vi "wifi-sub.vi"(0 "IP address":refnum<visa-resource-name>="COM13", 1 "send data":string, 5 "error in (no error)":errorcluster, 6 "port":i32, 7 "timeout (10sec)":u32=10000, 9 "data存盘":bool=TRUE, 10 "mode":T1(ring), 11 "Receive bytes one time":i32=1452) -> (15 "timeout?":bool=TRUE, 19 "error IO":errorcluster)   [LabVIEW 2023, in "wifi-interface.lvlib"]
uses:
  wifi-interface.lvlib
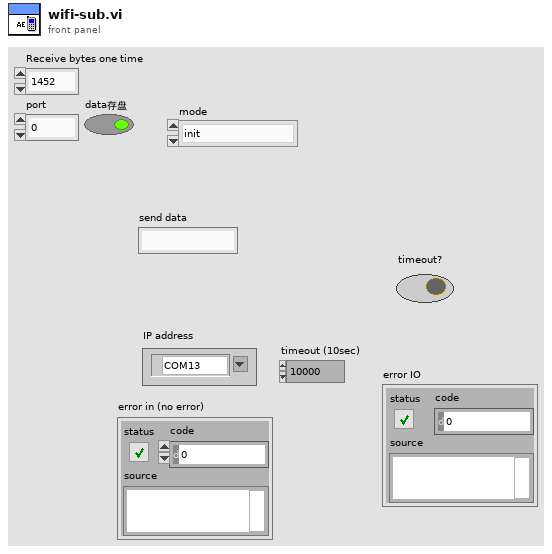
[diagram p1: front panel]
types:
  T1 = enum16{"init", "broadcast_data", "receive_data", "close", "clear_visa"}
  T2 = enum16{"Standard", "Buffered", "CRLF", "Immediate"}
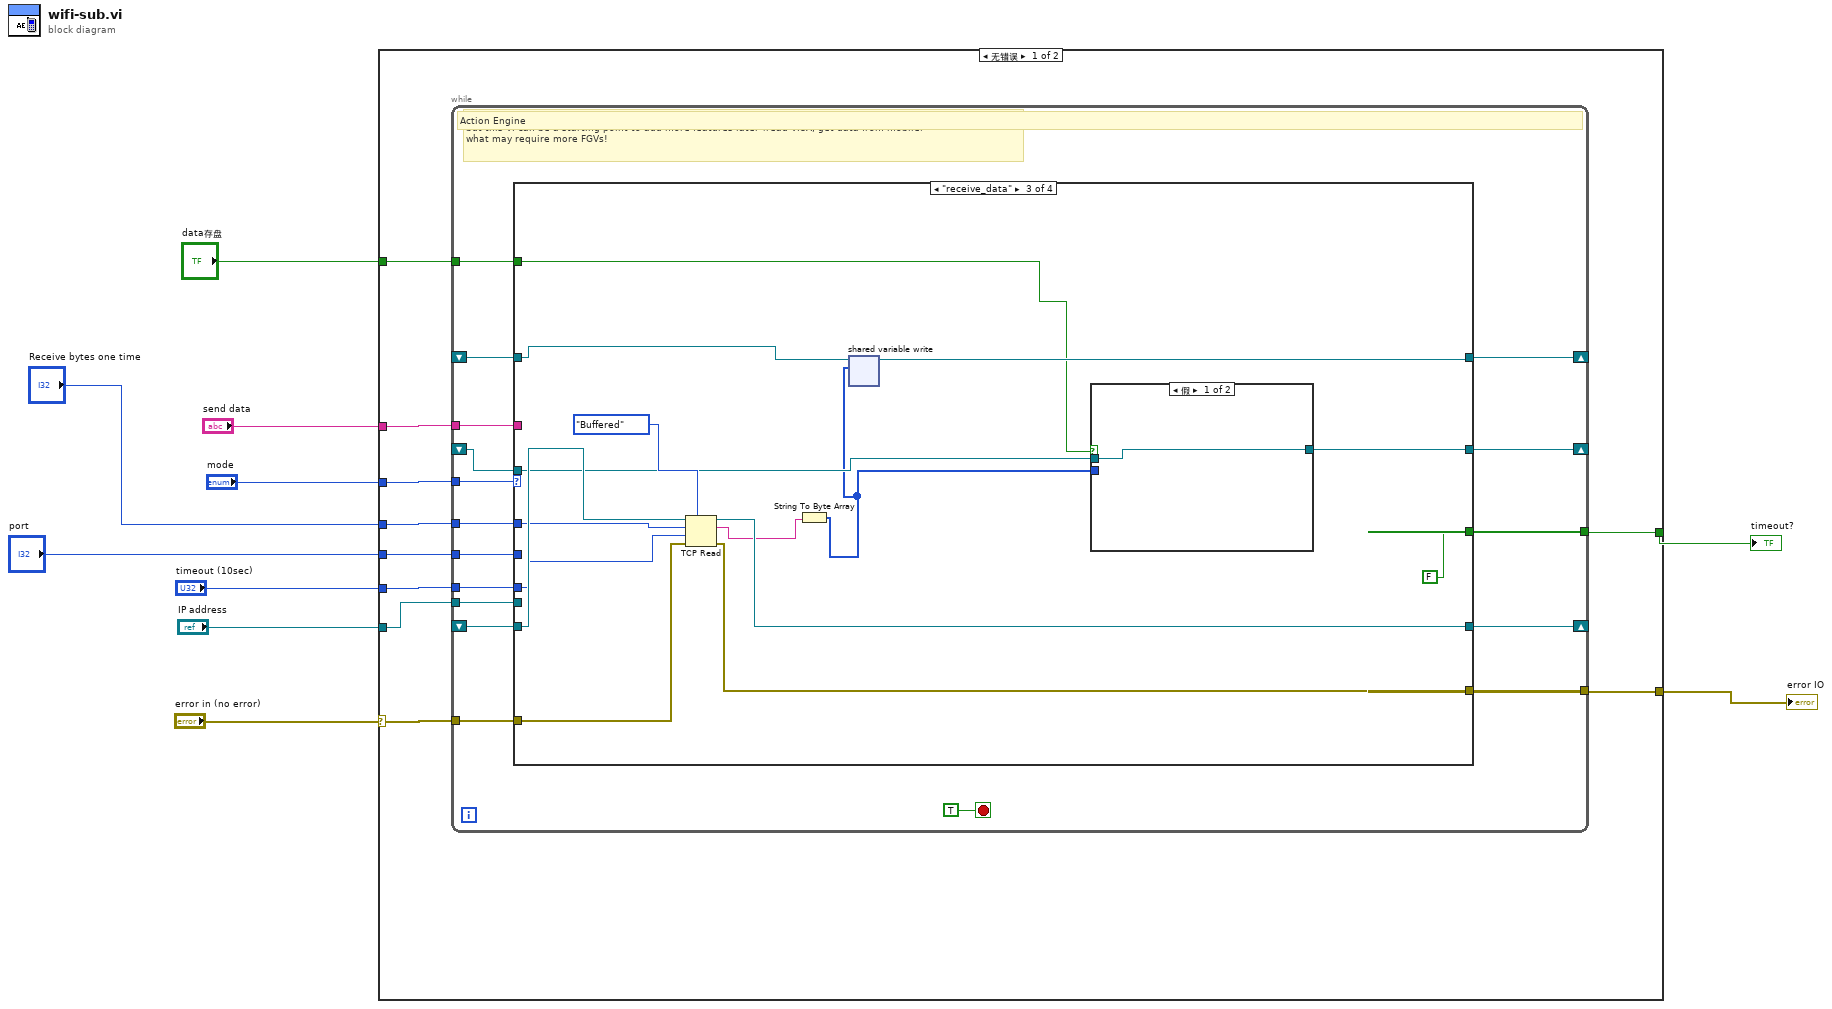
[diagram p0: block diagram]
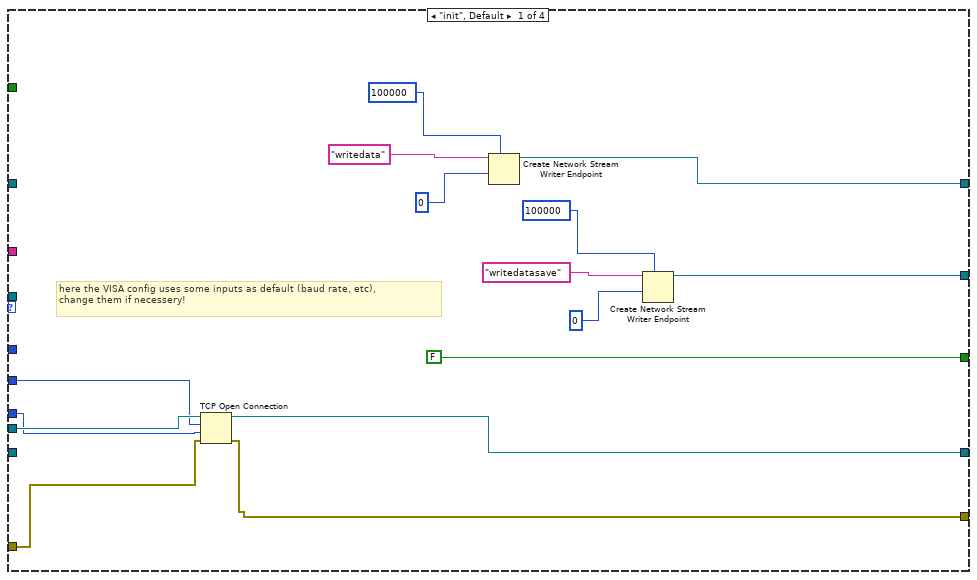
[diagram p2: hidden frame]
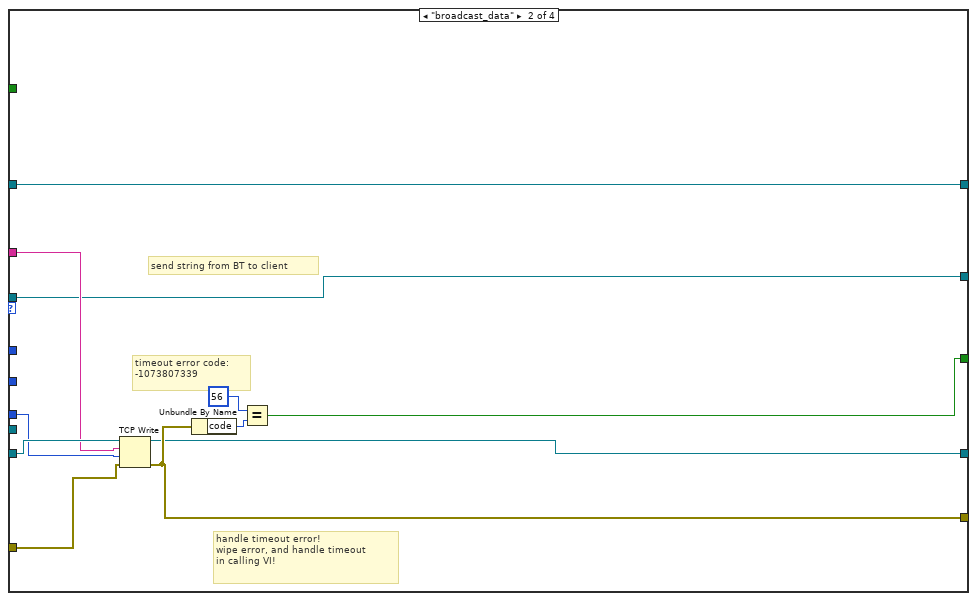
[diagram p3: hidden frame]
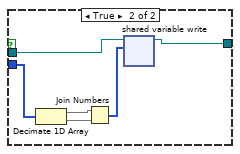
[diagram p4: hidden frame]
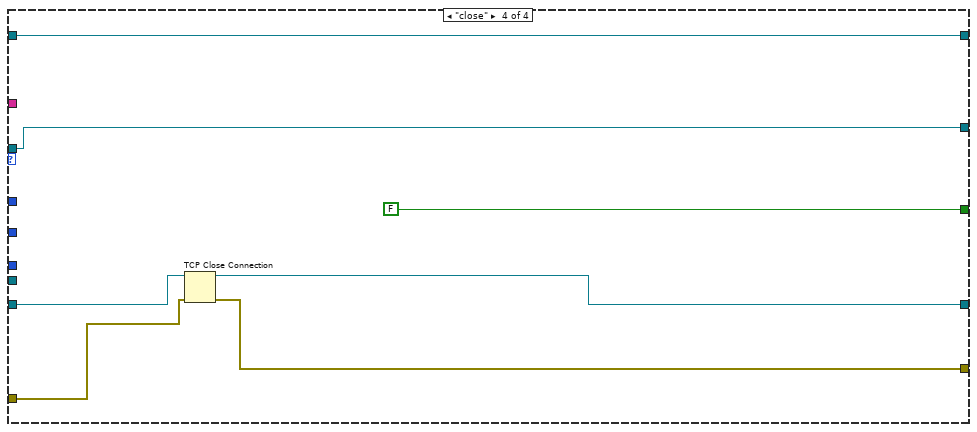
[diagram p5: hidden frame]
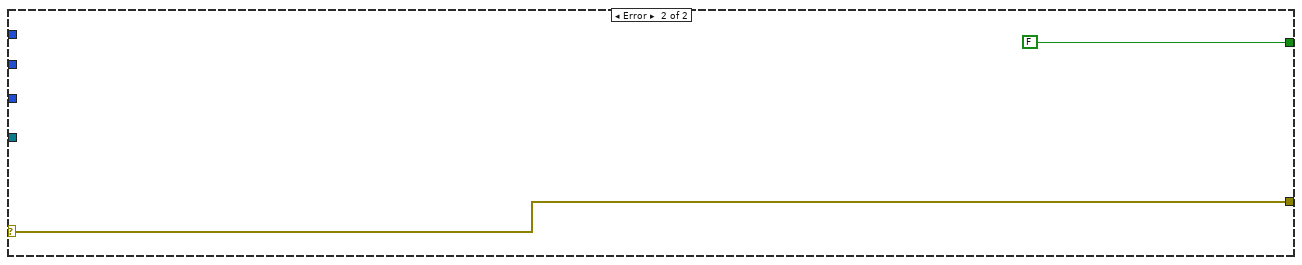
[diagram p6: hidden frame]
diagram:
  n1 = case shown="无错误" "error in (no error)" {
    selector: "error in (no error)" -> [w20 w94]
    tunnel: [w17 w94] -> w9
    tunnel: "mode" -> [w19 _]
    tunnel: "timeout (10sec)" -> [w18 _]
    tunnel: "IP address" -> [w14 _]
    tunnel: "send data" -> [w16 _]
    tunnel: [w15 FALSE] -> w4
    tunnel: "Receive bytes one time" -> [w13 _]
    tunnel: "port" -> [w12 _]
    tunnel: "data存盘" -> [w11 _]
    frame No Error {
      n2 = while {
        tunnel: w20 -> [w36]
        tunnel: w19 -> [w35]
        tunnel: w18 -> [w34]
        shift-right: [w33] -> _
        shift-left: _ -> [w28]
        tunnel: [w32] -> w17
        tunnel: w16 -> [w31]
        tunnel: [w30] -> w15
        tunnel: w14 -> [w29]
        tunnel: w13 -> [w27]
        tunnel: w12 -> [w26]
        tunnel: w11 -> [w25]
        shift-right: [w24] -> _
        shift-left: _ -> [w22]
        shift-right: [w23] -> _
        shift-left: _ -> [w21]
        stop <- TRUE stop-if-true
        # "actually this AE does have only 1 FGV yet, \nbut this VI can be a starting point to add more features later (read VISA, get data from mobile)\nwhat may require more FGVs!"
        # "Action Engine"
        n3 = case shown="\"receive_data\"" w35 {
          tunnel: w36 -> [w48 w57 w74 w88]
          tunnel: w34 -> [w49 w58 w73 _]
          tunnel: w29 -> [w51 _ _ _]
          tunnel: [w46 w55 w71 w90] -> w33
          tunnel: [w47 w56 w72 w89] -> w32
          tunnel: w31 -> [_ w59 _ _]
          tunnel: [FALSE w61 FALSE FALSE] -> w30
          tunnel: w28 -> [_ w60 w77 w91]
          tunnel: w27 -> [_ _ w75 _]
          tunnel: w26 -> [w50 _ _ _]
          tunnel: w25 -> [_ _ w67 _]
          tunnel: [w42 w54 w68 w87] -> w24
          tunnel: [w38 w53 w65 w86] -> w23
          tunnel: w22 -> [_ w54 w69 w87]
          tunnel: w21 -> [_ w53 w66 w86]
          frame "init", Default {
            # "here the VISA config uses some inputs as default (baud rate, etc),\nchange them if necessery!"
            n4 = TCP Open Connection(address=w51, remote port or service name=w50, timeout ms (60000)=w49, error in (no error)=w48) -> (connection ID=w46:refnum<k5>, error out=w47:errorcluster)  [unwired: 1 in]
            n5 = Create Network Stream Writer Endpoint(7:100000, 9:u8 0, 11:"writedata") -> (3:w42:refnum<k21>)  [unwired: 4 in, 1 out]
            n6 = Create Network Stream Writer Endpoint(7:100000, 9:u16 0, 11:"writedatasave") -> (3:w38:refnum<k21>)  [unwired: 4 in, 1 out]
          }
          frame "broadcast_data" {
            # "send string from BT to client"
            # "handle timeout error!\nwipe error, and handle timeout\nin calling VI!"
            # "timeout error code:\n-1073807339"
            n7 = TCP Write(connection ID=w60, data in=w59, error in (no error)=w57, 9:w58) -> (connection ID out=w55:refnum<k5>, error out=w56:errorcluster)  [unwired: 1 out]
            n8 = Unbundle By Name(w56) -> ("code"=w63:i32)
            n9 = Equal?(x=56 ("code"), y=w63) -> (x = y?=w61:bool)
          }
          frame "receive_data" {
            n10 = TCP Read(connection ID=w77, bytes to read=w75, error in (no error)=w74, 7:T2."Buffered" ("模式（标准）"), 9:w73) -> (connection ID out=w71:refnum<k5>, data out=w70:string, error out=w72:errorcluster)
            n11 = String To Byte Array(string=w70) -> (unsigned byte array=w64:u8[])
            n12 = shared-variable-write(w69, w64) -> (w68:refnum<k21>)  [unwired: 2 in, 2 out]
            n13 = case shown="假" w67 {
              tunnel: w66 -> [w79 w80]
              tunnel: [w79 w81] -> w65
              tunnel: w64 -> [_ w83]
              frame False {
              }
              frame True {
                n14 = Decimate 1D Array(w83) -> (w84:u8[], w85:u8[])
                n15 = Join Numbers(hi=w84, lo=w85) -> ((hi.lo)=w82:u16[])
                n16 = shared-variable-write(w80, w82) -> (w81:refnum<k21>)  [unwired: 2 in, 2 out]
              }
            }
          }
          frame "close" {
            n17 = TCP Close Connection(connection ID=w91, error in (no error)=w88) -> (connection ID out=w90:refnum<k5>, error out=w89:errorcluster)  [unwired: 1 in]
          }
        }
      }
    }
    frame Error {
    }
  }
  "error IO" <- w9
  "timeout?" <- w4
